vi "Read State.vi"(10 "result allocation in":T6, 11 "Sequencer Module runtime in":refnum<class "Sequencer Module runtime.lvclass">) -> (1 "State cluster":T1, 2 "result allocation out":T6, 3 "Sequencer Module runtime out":refnum<class "Sequencer Module runtime.lvclass">)   [LabVIEW 2015, in "Sequencer Module runtime.lvclass"]
uses:
  Sequencer Module runtime.lvclass
  <vilib>/NI/Tag Bus/table/data table.ctl
  Sequencer State Cluster.ctl
  Sequencer State Enum.ctl
  classes/Step/Execution/StepState.ctl
  classes/Step/Execution/Step Status.ctl
  classes/Step/Execution/Step Flow Control.ctl
  Sequencer Module runtime.lvclass/Sequencer Module runtime.ctl
  <vilib>/NI/Tag Bus/table/data polymorphs/read one/read I32.vi
  <vilib>/NI/Tag Bus/table/data polymorphs/read one/read String.vi
  <vilib>/NI/Tag Bus/table/data table.lvlib
  classes/Step/Execution/Step.lvclass
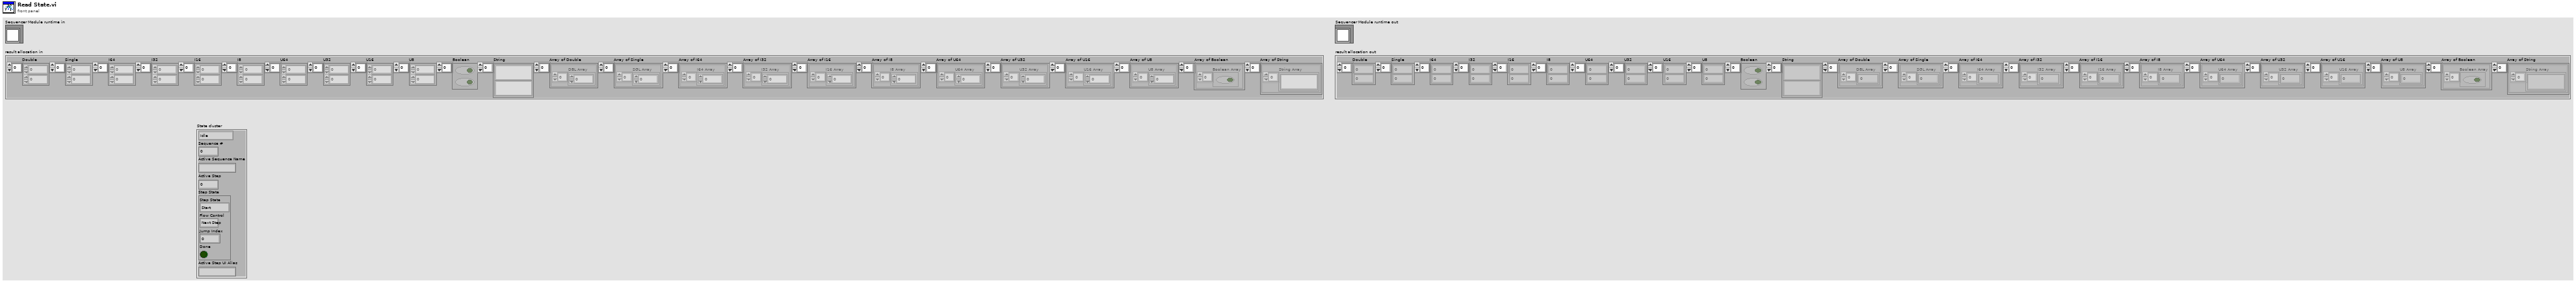
[diagram p1: front panel]
types:
  T1 = typedef "Sequencer Module runtime.lvclass/Sequencer State Cluster.ctl" = cluster{"Sequencer State":T2, "Sequence #":i32, "Active Sequence Name":string, "Active Step":i32, "Step State":T3, "Active Step UI Alias":string}
  T2 = typedef "Sequencer Module runtime.lvclass/Sequencer State Enum.ctl" = enum16{"Idle", "Paused", "Start Sequence", "Run Sequence", "CleanUp Sequence", "Generate Report"}
  T3 = typedef "Step.lvclass/StepState.ctl" = cluster{"Step State":T4, "Flow Control":T5, "Jump Index":i32, "Done":bool}
  T4 = typedef "Step.lvclass/Step Status.ctl" = enum16{"Start", "Passed", "Failed", "Error", "Done", "Terminated", "Skipped", "Running"}
  T5 = typedef "Step.lvclass/Step Flow Control.ctl" = enum16{"Next Step", "Jump"}
  T6 = typedef "tag bus.lvlib/data table.lvlib/data table.ctl" = cluster{"Double":dbl[], "Single":sgl[], "I64":i64[], "I32":i32[], "I16":i16[], "I8":i8[], "U64":u64[], "U32":u32[], "U16":u16[], "U8":u8[], "Boolean":bool[], "String":string[], "Array of Double":cluster{"DBL Array":dbl[]}[], "Array of Single":cluster{"SGL Array":sgl[]}[], "Array of I64":cluster{"I64 Array":i64[]}[], "Array of I32":cluster{"I32 Array":i32[]}[], "Array of I16":cluster{"I16 Array":i16[]}[], "Array of I8":cluster{"I8 Array":i8[]}[], "Array of U64":cluster{"U64 Array":u64[]}[], "Array of U32":cluster{"U32 Array":u32[]}[], "Array of U16":cluster{"U16 Array":u16[]}[], "Array of U8":cluster{"U8 Array":u8[]}[], "Array of Boolean":cluster{"Boolean Array":bool[]}[], "Array of String":cluster{"String Array":string[]}[]}
  T7 = typedef "Sequencer Module runtime.lvclass/Sequencer State Index.ctl" = cluster{"Sequencer State":i32, "Active Sequence Name":i32, "Active Sequence Index":i32, "Active Step":i32, "Active Step State":i32, "Active Step UI Alias":i32}
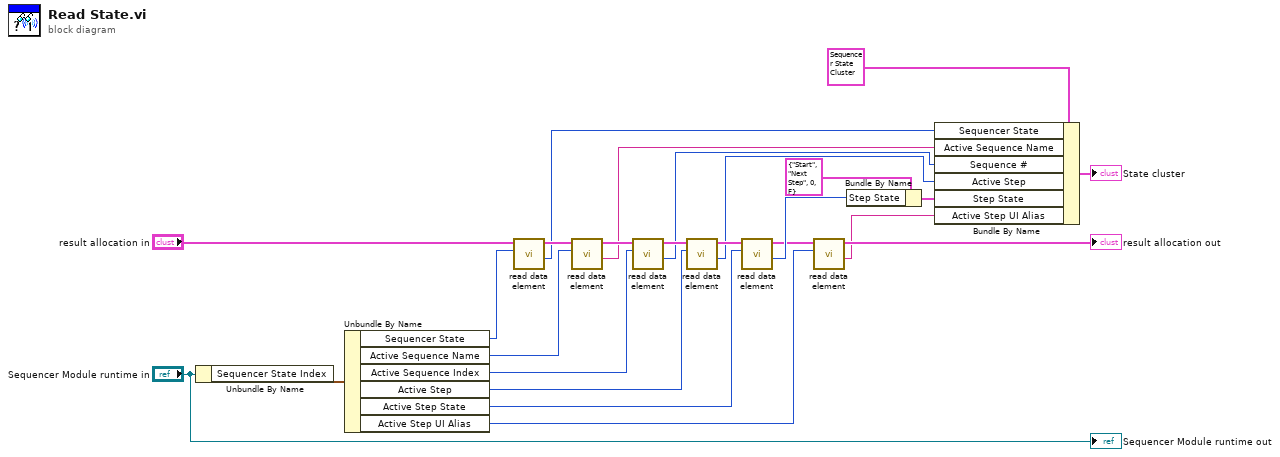
[diagram p0: block diagram]
diagram:
  n1 = Unbundle By Name("Sequencer Module runtime in") -> ("Sequencer State Index"=w24:T7)
  n2 = Unbundle By Name(w24) -> ("Sequencer State"=w22:i32, "Active Sequence Name"=w21:i32, "Active Sequence Index"=w20:i32, "Active Step"=w19:i32, "Active Step State"=w9:i32, "Active Step UI Alias"=w2:i32)
  n3 = call-poly <vilib>:"read data element.vi"("index"=w22, "data table in"="result allocation in") -> ("value"=w14:i32, "data table out"=w17:T6)  [unwired: 8 in]
  n4 = call-poly <vilib>:"read data element.vi"("index"=w21, "data table in"=w17) -> ("value"=w13:string, "data table out"=w16:T6)  [unwired: 8 in]
  n5 = call-poly <vilib>:"read data element.vi"("index"=w20, "data table in"=w16) -> ("value"=w12:i32, "data table out"=w15:T6)  [unwired: 8 in]
  n6 = call-poly <vilib>:"read data element.vi"("index"=w19, "data table in"=w15) -> ("value"=w5:i32, "data table out"=w10:T6)  [unwired: 8 in]
  n7 = call-poly <vilib>:"read data element.vi"("index"=w9, "data table in"=w10) -> ("value"=w7:i32, "data table out"=w4:T6)  [unwired: 8 in]
  n8 = call-poly <vilib>:"read data element.vi"("index"=w2, "data table in"=w4) -> ("value"=w1:string, "data table out"=→"result allocation out":T6)  [unwired: 8 in]
  n9 = Bundle By Name(cluster=T3 {"Step State"=enum."Start", "Flow Control"=enum."Next Step", "Jump Index"=0, "Done"=FALSE} ("Step State"), "Step State"=w7) -> (w6:T3)
  n10 = Bundle By Name(cluster=T1 {"Sequencer State"=enum."Idle", "Sequence #"=0, "Active Sequence Name"="", "Active Step"=0, "Step State"={"Step State"=enum."Start", "Flow Control"=enum."Next Step", "Jump Index"=0, "Done"=FALSE}, "Active Step UI Alias"=""} ("Sequencer State"), "Sequencer State"=w14, "Active Sequence Name"=w13, "Sequence #"=w12, "Active Step"=w5, "Step State"=w6, "Active Step UI Alias"=w1) -> (→"State cluster":T1)
  "Sequencer Module runtime out" <- "Sequencer Module runtime in"
